vi "Lights.vi"(8 "Input4":bool, 9 "Input3":bool, 10 "Input2":bool, 11 "Input1":bool) -> ()   [LabVIEW 2011]
uses:
  System Set Points and States.vi
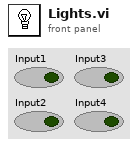
[diagram p1: front panel]
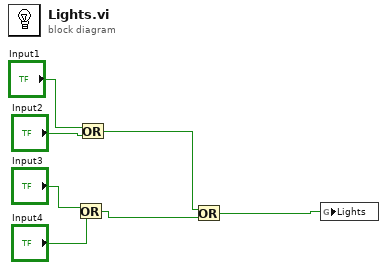
[diagram p0: block diagram]
diagram:
  n1 = Or(x="Input3", y="Input4") -> (x .or. y?=w6:bool)
  n2 = Or(x="Input1", y="Input2") -> (x .or. y?=w7:bool)
  n3 = Or(x=w7, y=w6) -> (x .or. y?=w1:bool)
  n4 = global write "System Set Points and States.vi" "Lights"(w1) -> ()
